vi "MainWindow.vi"() -> ()   [LabVIEW 2022 SP3]
panel:
  out "Luhn Calculation OK":bool=TRUE
  out "Valid \"Personnummer\"":bool=TRUE
  out "Luhn Number":string
  in  "Personal Number for calculation":string="640823-323"
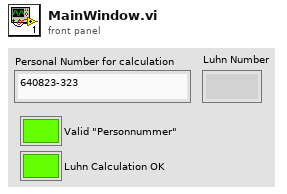
[diagram p1: front panel]
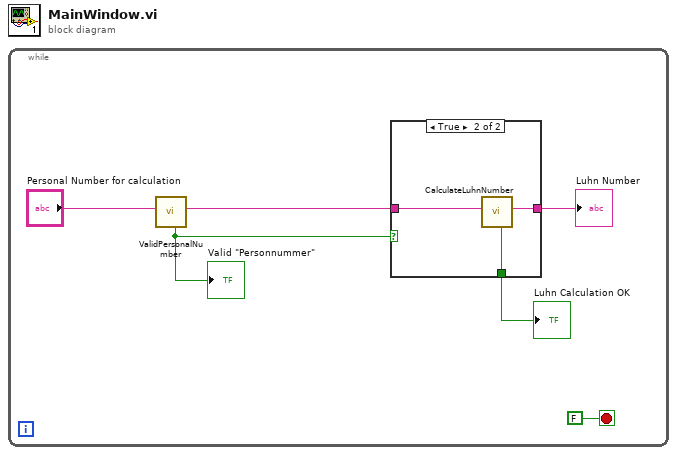
[diagram p0: block diagram]
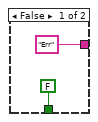
[diagram p2: hidden frame]
diagram:
  n1 = while {
    stop <- FALSE stop-if-true
    n2 = call "ValidPersonalNumber.vi"("InputString"="Personal Number for calculation") -> ("OutputString"=w4:string, "Valid?"=w1:bool)  [unwired: 9 in]
    "Valid \"Personnummer\"" <- w1
    n3 = case shown="True" w1 {
      tunnel: w4 -> [_ w11]
      tunnel: ["Err" ("String 2") w10] -> w3
      tunnel: [FALSE ("Valid") w9] -> w2
      frame False {
      }
      frame True {
        n4 = call "CalculateLuhnNumber.vi"("InputString"=w11) -> ("String 2"=w10:string, "Valid"=w9:bool)  [unwired: 9 in]
      }
    }
    "Luhn Number" <- w3
    "Luhn Calculation OK" <- w2
  }
